vi "Evaluate Part 2_2.vi"() -> ()   [LabVIEW 2020]
uses:
  Stateless Network/Stateless Network.lvclass
panel:
  out "Steps":u64[](array[numeric])
  in  "Input":string
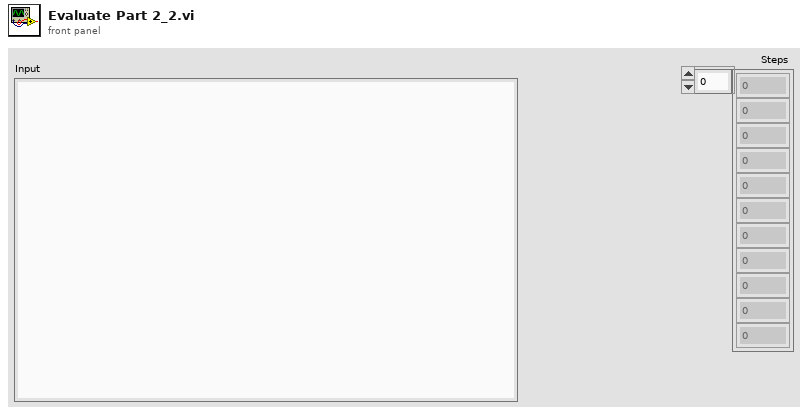
[diagram p1: front panel]
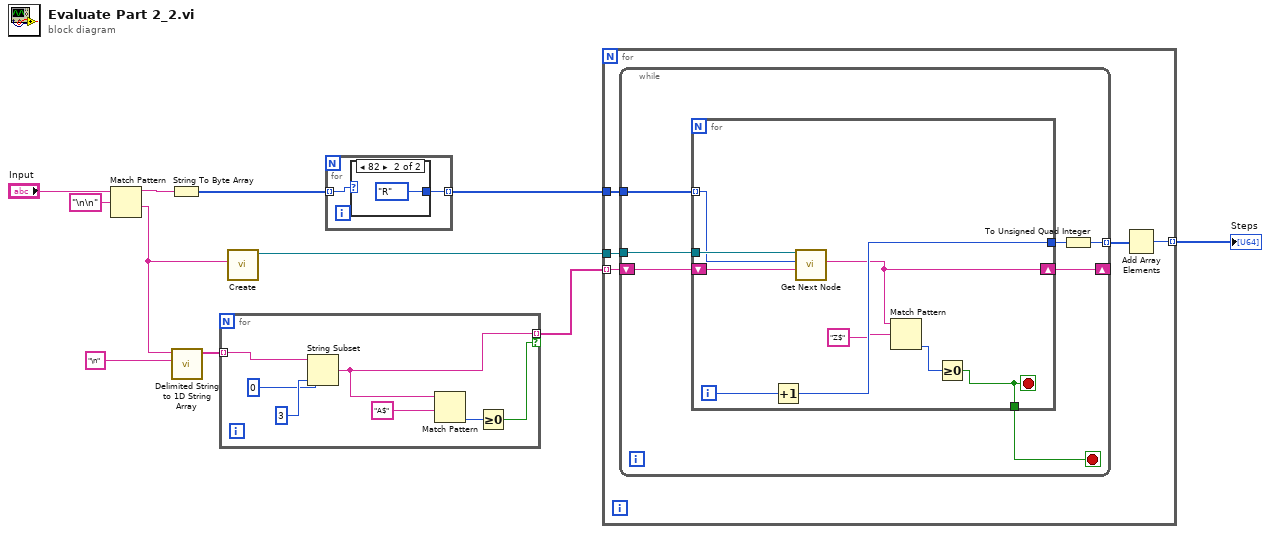
[diagram p0: block diagram]
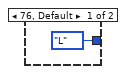
[diagram p2: hidden frame]
diagram:
  n1 = Match Pattern(string="Input", regular expression="\n\n" ("search string/char (-)")) -> (before substring=w9:string, after substring=w3:string)  [unwired: 1 in, 2 out]
  n2 = String To Byte Array(string=w9) -> (unsigned byte array=w8:u8[])
  n3 = call <vilib>:"Delimited String to 1D String Array.vi"("delimiter"="\n" ("search string/char (-)"), "delimited string"=w3) -> ("string array"=w4:string[])  [unwired: 9 in]
  n4 = for {
    tunnel: w4 -> [w13] mode=indexing
    tunnel: [w12] -> w2 mode=indexing if=w16
    n5 = String Subset(string=w13, offset (0)=0, length (rest)=3 ("length (rest)")) -> (substring=w12:string)
    n6 = Match Pattern(string=w12, regular expression="A$" ("y")) -> (offset past match=w17:i32)  [unwired: 1 in, 3 out]
    n7 = Greater Or Equal To 0?(x=w17) -> (x >= 0?=w16:bool)
  }
  n8 = call "Create.vi"("Input"=w3) -> ("Network"=w6:refnum<class "Stateless Network.lvclass">)  [unwired: 9 in, 1 out]
  n9 = for {
    tunnel: w8 -> [w20] mode=indexing
    tunnel: [w19] -> w7 mode=indexing
    n10 = case shown="82" w20 {
      tunnel: [enum16{"L", "R"}."L" ("Direction") enum16{"L", "R"}."R" ("Direction")] -> w19
      frame 76, Default {
      }
      frame 82 {
      }
    }
  }
  n11 = for {
    tunnel: w7 -> [w27]
    tunnel: w6 -> [w26]
    tunnel: w2 -> [w25] mode=indexing
    tunnel: [w23] -> w1 mode=indexing
    n12 = while {
      tunnel: w27 -> [w34]
      tunnel: [w30] -> w24 mode=indexing
      tunnel: w26 -> [w33]
      shift-right: [w28] -> _
      shift-left: w25 -> [w29]
      stop <- w31 stop-if-true
      n13 = for {
        tunnel: w34 -> [w42] mode=indexing
        tunnel: [w40] -> w32
        tunnel: [w37] -> w31
        tunnel: w33 -> [w43]
        shift-right: [w35] -> w28
        shift-left: w29 -> [w36]
        i -> [w41]
        stop <- w37 stop-if-true
        n14 = Increment(x=w41) -> (x+1=w40:i32)
        n15 = call "Get Next Node.vi"("State"=w36, "Direction"=w42, "Network in"=w43) -> ("Node"=w35:string)  [unwired: 6 in, 2 out]
        n16 = Match Pattern(string=w35, regular expression="Z$" ("y")) -> (offset past match=w38:i32)  [unwired: 1 in, 3 out]
        n17 = Greater Or Equal To 0?(x=w38) -> (x >= 0?=w37:bool)
      }
      n18 = To Unsigned Quad Integer(1:w32) -> (0:w30:u64)
    }
    n19 = Add Array Elements(numeric array=w24) -> (sum=w23:u64)
  }
  "Steps" <- w1
